vi "GeoData.vi"() -> ()   [LabVIEW 2017]
panel:
  out "StateFIPS":i32[](array[numeric])
  out "EINS":i32[](array[numeric])
  out "StateName":string[](array[string])
  out "County":string[](array[string])
  out "State":string[](array[string])
  out "City":string[](array[string])
  out "Fips":i32[](array[numeric])
  out "Zip":i32[](array[numeric])
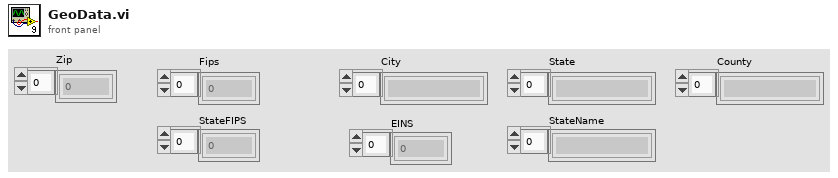
[diagram p1: front panel]
diagram:
  n1 = Spreadsheet String To Array(format string="%s", spreadsheet string="36091\t1001\tVerbena\tAL\tAutauga County\tH1\n36758\t1001\tPlantersville\tAL\tAutauga County\tH1\n36006\t1001\tBillingsley\tAL\tAutauga County\tH1\n36067\t1001\tPrattville\tAL\tAutauga County\tH1\n36701\t1001\tSelma\tAL\tAutauga County\tH1\n36003\t1001\tAutaugaville\tAL\tAutauga County\tH1\n36008\t1001\tBooth\tAL\tAutauga County\tH1\n36068\t1001\tPrattville\tAL\tAutauga County\tH1\n36022\t1001\tDeatsville\tAL\tAutauga County\tH1\n36703\t1001\tSelma\tAL\tAutauga County\tH1\n36749\t1001\tJones\tAL\tAutauga County\tH1\n36066\t1001\tPrattville\tAL\tAutauga County\tH1\n36051\t1001\tMarbury\tAL\tAutauga County\tH1\n36502\t1003\tAtmore\tAL\tBaldwin County\tH1\n36507\t1003\tBay minette\tAL\tBaldwin County\tH1\n36527\t1003\tDaphne\tAL\tBaldwin County\tH1\n36532\t1003\tFairhope\tAL\tBaldwin County\tH1\n36561\t1003\tOrange beach\tAL\tBaldwin County\tH1\n36550\t1003\tLittle river\tAL\tBaldwin County\tH1\n36564\t1003\tPoint clear\tAL\tBaldwin County\tH1\n36579\t1003\tStockton\tAL\tBaldwin County\tH1\n36526\t1003\tDaphne\tAL\tBaldwin County\tH1\n36551\t1003\tLoxley\tAL\tBaldwin County\tH1\n36555\t1003\tMagnolia springs\tAL\tBaldwin County\tH1\n36542\t1003\tGulf shores\tAL\tBaldwin County\tH1\n36567\t1003\tRobertsdale\tAL\tBaldwin County\tH1\n36533\t1003\tFairhope\tAL\tBaldwin County\tH1\n36576\t1003\tSilverhill\tAL\tBaldwin County\tH1\n36580\t1003\tSummerdale\tAL\tBaldwin County\tH1\n36547\t1003\tGulf shores\tAL\tBaldwin County\tH1\n36559\t1003\tMontrose\tAL\tBaldwin County\tH1\n36562\t1003\tPerdido\tAL\tBaldwin County\tH1\n36549\t1003\tLillian\tAL\tBaldwin County\tH1\n36577\t1003\tSpanish fort\tAL\tBaldwin County\tH1\n36511\t1003\tBon secour\tAL\tBaldwin County\tH1\n36530\t1003\tElberta\tAL\tBaldwin County\tH1\n36480\t1003\tUriah\tAL\tBaldwin County\tH1\n36535\t1003\tFoley\tAL\tBaldwin County\tH1\n36574\t1003\tSeminole\tAL\tBaldwin County\tH1\n36536\t1003\tFoley\tAL\tBaldwin County\tH1\n36578\t1003\tStapleton\tAL\tBaldwin County\tH1\n36017\t1005\tClio\tAL\tBarbour County\tH1\n36016\t1005\tClayton\tAL\tBarbour County\tH1\n36317\t1005\tClopton\tAL\tBarbour County\tH1\n36072\t1005\tEufaula\tAL\tBarbour County\tH1\n36311\t1005\tAriton\tAL\tBarbour County\tH1\n36048\t1005\tLouisville\tAL\tBarbour County\tH1\n36053\t1005\tMidway\tAL\tBarbour County\tH1\n36374\t1005\tSkipperville\tAL\tBarbour County\tH1\n36027\t1005\tEufaula\tAL\tBarbour County\tH1\n35115\t1007\tMontevallo\tAL\tBibb County\tH1\n35184\t1007\tWest blocton\tAL\tBibb County\tH1\n36750\t1007\tMaplesville\tAL\tBibb County\tH1\n36756\t1007\tMarion\tAL\tBibb County\tH1\n35074\t1007\tGreen pond\tAL\tBibb County\tH1\n35042\t1007\tCentreville\tAL\tBibb County\tH1\n35111\t1007\tMc calla\tAL\tBibb County\tH1\n35456\t1007\tDuncanville\tAL\tBibb County\tH1\n36792\t1007\tRandolph\tAL\tBibb County\tH1\n35080\t1007\tHelena\tAL\tBibb County\tH1\n35188\t1007\tWoodstock\tAL\tBibb County\tH1\n35034\t1007\tBrent\tAL\tBibb County\tH1\n35035\t1007\tBrierfield\tAL\tBibb County\tH1\n36793\t1007\tLawley\tAL\tBibb County\tH1\n35063\t1009\tEmpire\tAL\tBlount County\tH1\n35146\t1009\tSpringville\tAL\tBlount County\tH1\n35980\t1009\tHorton\tAL\tBlount County\tH1\n35013\t1009\tAllgood\tAL\tBlount County\tH1\n35126\t1009\tPinson\tAL\tBlount County\tH1\n35097\t1009\tLocust fork\tAL\tBlount County\tH1\n35049\t1009\tCleveland\tAL\tBlount County\tH1\n35172\t1009\tTrafford\tAL\tBlount County\tH1\n35957\t1009\tBoaz\tAL\tBlount County\tH1\n35031\t1009\tBlountsville\tAL\tBlount County\tH1\n35133\t1009\tRemlap\tAL\tBlount County\tH1\n35976\t1009\tGuntersville\tAL\tBlount County\tH1\n35016\t1009\tArab\tAL\tBlount County\tH1\n35121\t1009\tOneonta\tAL\tBlount County\tH1\n35079\t1009\tHayden\tAL\tBlount County\tH1\n35180\t1009\tWarrior\tAL\tBlount County\tH1\n35952\t1009\tAltoona\tAL\tBlount County\tH1\n36029\t1011\tFitzpatrick\tAL\tBullock County\tH1\n36052\t1011\tMathews\tAL\tBullock County\tH1\n36089\t1011\tUnion springs\tAL\tBullock County\tH1\n36860\t1011\tHurtsboro\tAL\tBullock County\tH1\n36031\t1011\tFort davis\tAL\tBullock County\tH1\n36081\t1011\tTroy\tAL\tBullock County\tH1\n36053\t1011\tMidway\tAL\tBullock County\tH1\n36005\t1011\tBanks\tAL\tBullock County\tH1\n36830\t1011\tAuburn\tAL\tBullock County\tH1\n36071\t1013\tRutledge\tAL\tButler County\tH1\n36015\t1013\tChapman\tAL\tButler County\tH1\n36042\t1013\tHonoraville\tAL\tButler County\tH1\n36474\t1013\tRed level\tAL\tButler County\tH1\n36033\t1013\tGeorgiana\tAL\tButler County\tH1\n36456\t1013\tMc kenzie\tAL\tButler County\tH1\n36030\t1013\tForest home\tAL\tButler County\tH1\n36032\t1013\tFort deposit\tAL\tButler County\tH1\n36037\t1013\tGreenville\tAL\tButler County\tH1\n36205\t1015\tAnniston\tAL\tCalhoun County\tH1\n36250\t1015\tAlexandria\tAL\tCalhoun County\tH1\n36204\t1015\tAnniston\tAL\tCalhoun County\tH1\n36253\t1015\tBynum\tAL\tCalhoun County\tH1\n35096\t1015\tLincoln\tAL\tCalhoun County\tH1\n35905\t1015\tGadsden\tAL\tCalhoun County\tH1\n36206\t1015\tAnniston\tAL\tCalhoun County\tH1\n36277\t1015\tWeaver\tAL\tCalhoun County\tH1\n36260\t1015\tEastaboga\tAL\tCalhoun County\tH1\n36207\t1015\tAnniston\tAL\tCalhoun County\tH1\n36272\t1015\tPiedmont\tAL\tCalhoun County\tH1\n36202\t1015\tAnniston\tAL\tCalhoun County\tH1\n36265\t1015\tJacksonville\tAL\tCalhoun County\tH1\n36201\t1015\tAnniston\tAL\tCalhoun County\tH1\n36203\t1015\tOxford\tAL\tCalhoun County\tH1\n36257\t1015\tDe armanville\tAL\tCalhoun County\tH1\n36271\t1015\tOhatchee\tAL\tCalhoun County\tH1\n36279\t1015\tWellington\tAL\tCalhoun County\tH1\n36254\t1015\tChoccolocco\tAL\tCalhoun County\tH1\n36854\t1017\tValley\tAL\tChambers County\tH1\n36850\t1017\tCamp hill\tAL\tChambers County\tH1\n36879\t1017\tWaverly\tAL\tChambers County\tH1\n36852\t1017\tCusseta\tAL\tChambers County\tH1\n36276\t1017\tWadley\tAL\tChambers County\tH1\n36274\t1017\tRoanoke\tAL\tChambers County\tH1\n36801\t1017\tOpelika\tAL\tChambers County\tH1\n36863\t1017\tLanett\tAL\tChambers County\tH1\n36862\t1017\tLafayette\tAL\tChambers County\tH1\n36855\t1017\tFive points\tAL\tChambers County\tH1\n35984\t1019\tMentone\tAL\tCherokee County\tH1\n35973\t1019\tGaylesville\tAL\tCherokee County\tH1\n35901\t1019\tGadsden\tAL\tCherokee County\tH1\n36275\t1019\tSpring garden\tAL\tCherokee County\tH1\n35903\t1019\tGadsden\tAL\tCherokee County\tH1\n35983\t1019\tLeesburg\tAL\tCherokee County\tH1\n35959\t1019\tCedar bluff\tAL\tCherokee County\tH1\n35961\t1019\tCollinsville\tAL\tCherokee County\tH1\n35967\t1019\tFort payne\tAL\tCherokee County\tH1\n36272\t1019\tPiedmont\tAL\tCherokee County\tH1\n35960\t1019\tCentre\tAL\tCherokee County\tH1\n35115\t1021\tMontevallo\tAL\tChilton County\tH1\n36091\t1021\tVerbena\tAL\tChilton County\tH1\n36758\t1021\tPlantersville\tAL\tChilton County\tH1\n36790\t1021\tStanton\tAL\tChilton County\tH1\n36006\t1021\tBillingsley\tAL\tChilton County\tH1\n36750\t1021\tMaplesville\tAL\tChilton County\tH1\n35045\t1021\tClanton\tAL\tChilton County\tH1\n36792\t1021\tRandolph\tAL\tChilton County\tH1\n35040\t1021\tCalera\tAL\tChilton County\tH1\n35046\t1021\tClanton\tAL\tChilton County\tH1\n35171\t1021\tThorsby\tAL\tChilton County\tH1\n36051\t1021\tMarbury\tAL\tChilton County\tH1\n35085\t1021\tJemison\tAL\tChilton County\tH1\n36793\t1021\tLawley\tAL\tChilton County\tH1\n36915\t1023\tNeedham\tAL\tChoctaw County\tH1\n36919\t1023\tSilas\tAL\tChoctaw County\tH1\n36910\t1023\tJachin\tAL\tChoctaw County\tH1\n36916\t1023\tPennington\tAL\tChoctaw County\tH1\n36908\t1023\tGilbertown\tAL\tChoctaw County\tH1\n36913\t1023\tMelvin\tAL\tChoctaw County\tH1\n36912\t1023\tLisman\tAL\tChoctaw County\tH1\n36921\t1023\tToxey\tAL\tChoctaw County\tH1\n36558\t1023\tMillry\tAL\tChoctaw County\tH1\n36904\t1023\tButler\tAL\tChoctaw County\tH1\n36922\t1023\tWard\tAL\tChoctaw County\tH1\n36540\t1025\tGainestown\tAL\tClarke County\tH1\n36524\t1025\tCoffeeville\tAL\tClarke County\tH1\n36751\t1025\tLower peach tree\tAL\tClarke County\tH1\n36727\t1025\tCampbell\tAL\tClarke County\tH1\n36545\t1025\tJackson\tAL\tClarke County\tH1\n36446\t1025\tFulton\tAL\tClarke County\tH1\n36451\t1025\tGrove hill\tAL\tClarke County\tH1\n36436\t1025\tDickinson\tAL\tClarke County\tH1\n36784\t1025\tThomasville\tAL\tClarke County\tH1\n36482\t1025\tWhatley\tAL\tClarke County\tH1\n36251\t1027\tAshland\tAL\tClay County\tH1\n35089\t1027\tKellyton\tAL\tClay County\tH1\n36266\t1027\tLineville\tAL\tClay County\tH1\n36267\t1027\tMillerville\tAL\tClay County\tH1\n36256\t1027\tDaviston\tAL\tClay County\tH1\n36258\t1027\tDelta\tAL\tClay County\tH1\n36255\t1027\tCragford\tAL\tClay County\tH1\n35072\t1027\tGoodwater\tAL\tClay County\tH1\n35160\t1027\tTalladega\tAL\tClay County\tH1\n36276\t1027\tWadley\tAL\tClay County\tH1\n36268\t1027\tMunford\tAL\tClay County\tH1\n35082\t1027\tHollins\tAL\tClay County\tH1\n36264\t1029\tHeflin\tAL\tCleburne County\tH1\n36269\t1029\tMuscadine\tAL\tCleburne County\tH1\n36258\t1029\tDelta\tAL\tCleburne County\tH1\n36207\t1029\tAnniston\tAL\tCleburne County\tH1\n36272\t1029\tPiedmont\tAL\tCleburne County\tH1\n36262\t1029\tFruithurst\tAL\tCleburne County\tH1\n36273\t1029\tRanburne\tAL\tCleburne County\tH1\n36261\t1029\tEdwardsville\tAL\tCleburne County\tH1\n36268\t1029\tMunford\tAL\tCleburne County\tH1\n36323\t1031\tElba\tAL\tCoffee County\tH1\n36360\t1031\tOzark\tAL\tCoffee County\tH1\n36079\t1031\tTroy\tAL\tCoffee County\tH1\n36322\t1031\tDaleville\tAL\tCoffee County\tH1\n36311\t1031\tAriton\tAL\tCoffee County\tH1\n36453\t1031\tKinston\tAL\tCoffee County\tH1\n36009\t1031\tBrantley\tAL\tCoffee County\tH1\n36351\t1031\tNew brockton\tAL\tCoffee County\tH1\n36010\t1031\tBrundidge\tAL\tCoffee County\tH1\n36330\t1031\tEnterprise\tAL\tCoffee County\tH1\n36316\t1031\tChancellor\tAL\tCoffee County\tH1\n36034\t1031\tGlenwood\tAL\tCoffee County\tH1\n36467\t1031\tOpp\tAL\tCoffee County\tH1\n36346\t1031\tJack\tAL\tCoffee County\tH1\n36477\t1031\tSamson\tAL\tCoffee County\tH1\n36318\t1031\tCoffee springs\tAL\tCoffee County\tH1\n35672\t1033\tTown creek\tAL\tColbert County\tH1\n35646\t1033\tLeighton\tAL\tColbert County\tH1\n35616\t1033\tCherokee\tAL\tColbert County\tH1\n35661\t1033\tMuscle shoals\tAL\tColbert County\tH1\n35674\t1033\tTuscumbia\tAL\tColbert County\tH1\n35654\t1033\tRussellville\tAL\tColbert County\tH1\n35660\t1033\tSheffield\tAL\tColbert County\tH1\n35653\t1033\tRussellville\tAL\tColbert County\tH1\n35582\t1033\tRed bay\tAL\tColbert County\tH1\n36502\t1035\tAtmore\tAL\tConecuh County\tH1\n36474\t1035\tRed level\tAL\tConecuh County\tH1\n36033\t1035\tGeorgiana\tAL\tConecuh County\tH1\n36456\t1035\tMc kenzie\tAL\tConecuh County\tH1\n36473\t1035\tRange\tAL\tConecuh County\tH1\n36330\t1035\tEnterprise\tAL\tConecuh County\tH1\n36471\t1035\tPeterman\tAL\tConecuh County\tH1\n36454\t1035\tLenox\tAL\tConecuh County\tH1\n36460\t1035\tMonroeville\tAL\tConecuh County\tH1\n36401\t1035\tEvergreen\tAL\tConecuh County\tH1\n36421\t1035\tAndalusia\tAL\tConecuh County\tH1\n36426\t1035\tBrewton\tAL\tConecuh County\tH1\n36432\t1035\tCastleberry\tAL\tConecuh County\tH1\n36475\t1035\tRepton\tAL\tConecuh County\tH1\n36768\t1035\tPine apple\tAL\tConecuh County\tH1\n35151\t1037\tSylacauga\tAL\tCoosa County\tH1\n35010\t1037\tAlexander city\tAL\tCoosa County\tH1\n35183\t1037\tWeogufka\tAL\tCoosa County\tH1\n35089\t1037\tKellyton\tAL\tCoosa County\tH1\n36026\t1037\tEquality\tAL\tCoosa County\tH1\n35150\t1037\tSylacauga\tAL\tCoosa County\tH1\n35072\t1037\tGoodwater\tAL\tCoosa County\tH1\n35136\t1037\tRockford\tAL\tCoosa County\tH1\n35046\t1037\tClanton\tAL\tCoosa County\tH1\n36080\t1037\tTitus\tAL\tCoosa County\tH1\n36476\t1039\tRiver falls\tAL\tCovington County\tH1\n36028\t1039\tDozier\tAL\tCovington County\tH1\n36474\t1039\tRed level\tAL\tCovington County\tH1\n36453\t1039\tKinston\tAL\tCovington County\tH1\n36456\t1039\tMc kenzie\tAL\tCovington County\tH1\n36038\t1039\tGantt\tAL\tCovington County\tH1\n36442\t1039\tFlorala\tAL\tCovington County\tH1\n36455\t1039\tLockhart\tAL\tCovington County\tH1\n36420\t1039\tAndalusia\tAL\tCovington County\tH1\n36401\t1039\tEvergreen\tAL\tCovington County\tH1\n36421\t1039\tAndalusia\tAL\tCovington County\tH1\n36467\t1039\tOpp\tAL\tCovington County\tH1\n36483\t1039\tWing\tAL\tCovington County\tH1\n36477\t1039\tSamson\tAL\tCovington County\tH1\n36323\t1041\tElba\tAL\tCrenshaw County\tH1\n36028\t1041\tDozier\tAL\tCrenshaw County\tH1\n36071\t1041\tRutledge\tAL\tCrenshaw County\tH1\n36042\t1041\tHonoraville\tAL\tCrenshaw County\tH1\n36009\t1041\tBrantley\tAL\tCrenshaw County\tH1\n36049\t1041\tLuverne\tAL\tCrenshaw County\tH1\n36041\t1041\tHighland home\tAL\tCrenshaw County\tH1\n36032\t1041\tFort deposit\tAL\tCrenshaw County\tH1\n36034\t1041\tGlenwood\tAL\tCrenshaw County\tH1\n36035\t1041\tGoshen\tAL\tCrenshaw County\tH1\n36467\t1041\tOpp\tAL\tCrenshaw County\tH1\n36037\t1041\tGreenville\tAL\tCrenshaw County\tH1\n36036\t1041\tGrady\tAL\tCrenshaw County\tH1\n36046\t1041\tLapine\tAL\tCrenshaw County\tH1\n35619\t1043\tDanville\tAL\tCullman County\tH1\n35541\t1043\tArley\tAL\tCullman County\tH1\n35057\t1043\tCullman\tAL\tCullman County\tH1\n35033\t1043\tBremen\tAL\tCullman County\tH1\n35055\t1043\tCullman\tAL\tCullman County\tH1\n35058\t1043\tCullman\tAL\tCullman County\tH1\n35077\t1043\tHanceville\tAL\tCullman County\tH1\n35070\t1043\tGarden city\tAL\tCullman County\tH1\n35087\t1043\tJoppa\tAL\tCullman County\tH1\n35083\t1043\tHolly pond\tAL\tCullman County\tH1\n35098\t1043\tLogan\tAL\tCullman County\tH1\n35976\t1043\tGuntersville\tAL\tCullman County\tH1\n35056\t1043\tCullman\tAL\tCullman County\tH1\n35053\t1043\tCrane hill\tAL\tCullman County\tH1\n35019\t1043\tBaileyton\tAL\tCullman County\tH1\n35016\t1043\tArab\tAL\tCullman County\tH1\n35179\t1043\tVinemont\tAL\tCullman County\tH1\n35540\t1043\tAddison\tAL\tCullman County\tH1\n35621\t1043\tEva\tAL\tCullman County\tH1\n35622\t1043\tFalkville\tAL\tCullman County\tH1\n35670\t1043\tSomerville\tAL\tCullman County\tH1\n36360\t1045\tOzark\tAL\tDale County\tH1\n36317\t1045\tClopton\tAL\tDale County\tH1\n36322\t1045\tDaleville\tAL\tDale County\tH1\n36361\t1045\tOzark\tAL\tDale County\tH1\n36371\t1045\tPinckard\tAL\tDale County\tH1\n36311\t1045\tAriton\tAL\tDale County\tH1\n36362\t1045\tFort rucker\tAL\tDale County\tH1\n36345\t1045\tHeadland\tAL\tDale County\tH1\n36010\t1045\tBrundidge\tAL\tDale County\tH1\n36330\t1045\tEnterprise\tAL\tDale County\tH1\n36352\t1045\tNewton\tAL\tDale County\tH1\n36374\t1045\tSkipperville\tAL\tDale County\tH1\n36303\t1045\tDothan\tAL\tDale County\tH1\n36353\t1045\tNewville\tAL\tDale County\tH1\n36350\t1045\tMidland city\tAL\tDale County\tH1\n36758\t1047\tPlantersville\tAL\tDallas County\tH1\n36773\t1047\tSafford\tAL\tDallas County\tH1\n36701\t1047\tSelma\tAL\tDallas County\tH1\n36785\t1047\tTyler\tAL\tDallas County\tH1\n36703\t1047\tSelma\tAL\tDallas County\tH1\n36775\t1047\tSardis\tAL\tDallas County\tH1\n36761\t1047\tMinter\tAL\tDallas County\tH1\n36749\t1047\tJones\tAL\tDallas County\tH1\n36767\t1047\tOrrville\tAL\tDallas County\tH1\n36759\t1047\tMarion junction\tAL\tDallas County\tH1\n35968\t1049\tFort payne\tAL\tDeKalb County\tH1\n35984\t1049\tMentone\tAL\tDeKalb County\tH1\n35765\t1049\tPisgah\tAL\tDeKalb County\tH1\n35954\t1049\tAttalla\tAL\tDeKalb County\tH1\n35983\t1049\tLeesburg\tAL\tDeKalb County\tH1\n35966\t1049\tFlat rock\tAL\tDeKalb County\tH1\n35975\t1049\tGroveoak\tAL\tDeKalb County\tH1\n35957\t1049\tBoaz\tAL\tDeKalb County\tH1\n35959\t1049\tCedar bluff\tAL\tDeKalb County\tH1\n35978\t1049\tHenagar\tAL\tDeKalb County\tH1\n35988\t1049\tSylvania\tAL\tDeKalb County\tH1\n35951\t1049\tAlbertville\tAL\tDeKalb County\tH1\n35961\t1049\tCollinsville\tAL\tDeKalb County\tH1\n35967\t1049\tFort payne\tAL\tDeKalb County\tH1\n35956\t1049\tBoaz\tAL\tDeKalb County\tH1\n35981\t1049\tIder\tAL\tDeKalb County\tH1\n35974\t1049\tGeraldine\tAL\tDeKalb County\tH1\n35979\t1049\tHigdon\tAL\tDeKalb County\tH1\n35989\t1049\tValley head\tAL\tDeKalb County\tH1\n35963\t1049\tDawson\tAL\tDeKalb County\tH1\n35962\t1049\tCrossville\tAL\tDeKalb County\tH1\n35971\t1049\tFyffe\tAL\tDeKalb County\tH1\n35986\t1049\tRainsville\tAL\tDeKalb County\tH1\n35771\t1049\tSection\tAL\tDeKalb County\tH1\n36024\t1051\tEclectic\tAL\tElmore County\tH1\n35010\t1051\tAlexander city\tAL\tElmore County\tH1\n36078\t1051\tTallassee\tAL\tElmore County\tH1\n36067\t1051\tPrattville\tAL\tElmore County\tH1\n36092\t1051\tWetumpka\tAL\tElmore County\tH1\n36093\t1051\tWetumpka\tAL\tElmore County\tH1\n36026\t1051\tEquality\tAL\tElmore County\tH1\n36054\t1051\tMillbrook\tAL\tElmore County\tH1\n35136\t1051\tRockford\tAL\tElmore County\tH1\n36025\t1051\tElmore\tAL\tElmore County\tH1\n36022\t1051\tDeatsville\tAL\tElmore County\tH1\n36066\t1051\tPrattville\tAL\tElmore County\tH1\n36051\t1051\tMarbury\tAL\tElmore County\tH1\n36020\t1051\tCoosada\tAL\tElmore County\tH1\n36080\t1051\tTitus\tAL\tElmore County\tH1\n36502\t1053\tAtmore\tAL\tEscambia County\tH1\n36441\t1053\tFlomaton\tAL\tEscambia County\tH1\n36420\t1053\tAndalusia\tAL\tEscambia County\tH1\n36426\t1053\tBrewton\tAL\tEscambia County\tH1\n36432\t1053\tCastleberry\tAL\tEscambia County\tH1\n36475\t1053\tRepton\tAL\tEscambia County\tH1\n36483\t1053\tWing\tAL\tEscambia County\tH1\n36562\t1053\tPerdido\tAL\tEscambia County\tH1\n36543\t1053\tHuxford\tAL\tEscambia County\tH1\n36503\t1053\tAtmore\tAL\tEscambia County\tH1\n35901\t1055\tGadsden\tAL\tEtowah County\tH1\n35954\t1055\tAttalla\tAL\tEtowah County\tH1\n35903\t1055\tGadsden\tAL\tEtowah County\tH1\n35907\t1055\tGadsden\tAL\tEtowah County\tH1\n35905\t1055\tGadsden\tAL\tEtowah County\tH1\n35904\t1055\tGadsden\tAL\tEtowah County\tH1\n35957\t1055\tBoaz\tAL\tEtowah County\tH1\n35961\t1055\tCollinsville\tAL\tEtowah County\tH1\n35972\t1055\tGallant\tAL\tEtowah County\tH1\n35956\t1055\tBoaz\tAL\tEtowah County\tH1\n36272\t1055\tPiedmont\tAL\tEtowah County\tH1\n35902\t1055\tGadsden\tAL\tEtowah County\tH1\n35990\t1055\tWalnut grove\tAL\tEtowah County\tH1\n35121\t1055\tOneonta\tAL\tEtowah County\tH1\n35952\t1055\tAltoona\tAL\tEtowah County\tH1\n35906\t1055\tRainbow city\tAL\tEtowah County\tH1\n36271\t1055\tOhatchee\tAL\tEtowah County\tH1\n35554\t1057\tEldridge\tAL\tFayette County\tH1\n35594\t1057\tWinfield\tAL\tFayette County\tH1\n35546\t1057\tBerry\tAL\tFayette County\tH1\n35549\t1057\tCarbon hill\tAL\tFayette County\tH1\n35579\t1057\tOakman\tAL\tFayette County\tH1\n35563\t1057\tGuin\tAL\tFayette County\tH1\n35542\t1057\tBankston\tAL\tFayette County\tH1\n35545\t1057\tBelk\tAL\tFayette County\tH1\n35574\t1057\tKennedy\tAL\tFayette County\tH1\n35555\t1057\tFayette\tAL\tFayette County\tH1\n35559\t1057\tGlen allen\tAL\tFayette County\tH1\n35585\t1059\tSpruce pine\tAL\tFranklin County\tH1\n35593\t1059\tVina\tAL\tFranklin County\tH1\n35581\t1059\tPhil campbell\tAL\tFranklin County\tH1\n35616\t1059\tCherokee\tAL\tFranklin County\tH1\n35674\t1059\tTuscumbia\tAL\tFranklin County\tH1\n35565\t1059\tHaleyville\tAL\tFranklin County\tH1\n35564\t1059\tHackleburg\tAL\tFranklin County\tH1\n35651\t1059\tMount hope\tAL\tFranklin County\tH1\n35654\t1059\tRussellville\tAL\tFranklin County\tH1\n35571\t1059\tHodges\tAL\tFranklin County\tH1\n35653\t1059\tRussellville\tAL\tFranklin County\tH1\n35582\t1059\tRed bay\tAL\tFranklin County\tH1\n36305\t1061\tDothan\tAL\tGeneva County\tH1\n36314\t1061\tBlack\tAL\tGeneva County\tH1\n36322\t1061\tDaleville\tAL\tGeneva County\tH1\n36375\t1061\tSlocomb\tAL\tGeneva County\tH1\n36453\t1061\tKinston\tAL\tGeneva County\tH1\n36340\t1061\tGeneva\tAL\tGeneva County\tH1\n36344\t1061\tHartford\tAL\tGeneva County\tH1\n36316\t1061\tChancellor\tAL\tGeneva County\tH1\n36442\t1061\tFlorala\tAL\tGeneva County\tH1\n36352\t1061\tNewton\tAL\tGeneva County\tH1\n36301\t1061\tDothan\tAL\tGeneva County\tH1\n36467\t1061\tOpp\tAL\tGeneva County\tH1\n36349\t1061\tMalvern\tAL\tGeneva County\tH1\n36477\t1061\tSamson\tAL\tGeneva County\tH1\n36318\t1061\tCoffee springs\tAL\tGeneva County\tH1\n36313\t1061\tBellwood\tAL\tGeneva County\tH1\n35480\t1063\tRalph\tAL\tGreene County\tH1\n35448\t1063\tClinton\tAL\tGreene County\tH1\n35464\t1063\tGainesville\tAL\tGreene County\tH1\n35443\t1063\tBoligee\tAL\tGreene County\tH1\n35463\t1063\tFosters\tAL\tGreene County\tH1\n35469\t1063\tKnoxville\tAL\tGreene County\tH1\n35491\t1063\tWest greene\tAL\tGreene County\tH1\n35462\t1063\tEutaw\tAL\tGreene County\tH1\n36740\t1063\tForkland\tAL\tGreene County\tH1\n36744\t1065\tGreensboro\tAL\tHale County\tH1\n36786\t1065\tUniontown\tAL\tHale County\tH1\n36756\t1065\tMarion\tAL\tHale County\tH1\n36765\t1065\tNewbern\tAL\tHale County\tH1\n35441\t1065\tAkron\tAL\tHale County\tH1\n35474\t1065\tMoundville\tAL\tHale County\tH1\n36742\t1065\tGallion\tAL\tHale County\tH1\n36776\t1065\tSawyerville\tAL\tHale County\tH1\n36738\t1065\tFaunsdale\tAL\tHale County\tH1\n36317\t1067\tClopton\tAL\tHenry County\tH1\n36373\t1067\tShorterville\tAL\tHenry County\tH1\n36319\t1067\tColumbia\tAL\tHenry County\tH1\n36345\t1067\tHeadland\tAL\tHenry County\tH1\n36303\t1067\tDothan\tAL\tHenry County\tH1\n36310\t1067\tAbbeville\tAL\tHenry County\tH1\n36353\t1067\tNewville\tAL\tHenry County\tH1\n36350\t1067\tMidland city\tAL\tHenry County\tH1\n36320\t1069\tCottonwood\tAL\tHouston County\tH1\n36305\t1069\tDothan\tAL\tHouston County\tH1\n36312\t1069\tAshford\tAL\tHouston County\tH1\n36375\t1069\tSlocomb\tAL\tHouston County\tH1\n36319\t1069\tColumbia\tAL\tHouston County\tH1\n36345\t1069\tHeadland\tAL\tHouston County\tH1\n36376\t1069\tWebb\tAL\tHouston County\tH1\n36352\t1069\tNewton\tAL\tHouston County\tH1\n36302\t1069\tDothan\tAL\tHouston County\tH1\n36301\t1069\tDothan\tAL\tHouston County\tH1\n36303\t1069\tDothan\tAL\tHouston County\tH1\n36321\t1069\tCowarts\tAL\tHouston County\tH1\n36343\t1069\tGordon\tAL\tHouston County\tH1\n36370\t1069\tPansey\tAL\tHouston County\tH1\n36350\t1069\tMidland city\tAL\tHouston County\tH1\n35751\t1071\tHollytree\tAL\tJackson County\tH1\n35752\t1071\tHollywood\tAL\tJackson County\tH1\n35765\t1071\tPisgah\tAL\tJackson County\tH1\n35745\t1071\tEstillfork\tAL\tJackson County\tH1\n35776\t1071\tWoodville\tAL\tJackson County\tH1\n35966\t1071\tFlat rock\tAL\tJackson County\tH1\n35769\t1071\tScottsboro\tAL\tJackson County\tH1\n35978\t1071\tHenagar\tAL\tJackson County\tH1\n35772\t1071\tStevenson\tAL\tJackson County\tH1\n35768\t1071\tScottsboro\tAL\tJackson County\tH1\n35748\t1071\tGurley\tAL\tJackson County\tH1\n35774\t1071\tTrenton\tAL\tJackson County\tH1\n35958\t1071\tBryant\tAL\tJackson County\tH1\n35740\t1071\tBridgeport\tAL\tJackson County\tH1\n35766\t1071\tPrinceton\tAL\tJackson County\tH1\n35979\t1071\tHigdon\tAL\tJackson County\tH1\n35744\t1071\tDutton\tAL\tJackson County\tH1\n35764\t1071\tPaint rock\tAL\tJackson County\tH1\n35971\t1071\tFyffe\tAL\tJackson County\tH1\n35746\t1071\tFackler\tAL\tJackson County\tH1\n35755\t1071\tLangston\tAL\tJackson County\tH1\n35771\t1071\tSection\tAL\tJackson County\tH1\n35022\t1073\tBessemer\tAL\tJefferson County\tH1\n35130\t1073\tQuinton\tAL\tJefferson County\tH1\n35208\t1073\tBirmingham\tAL\tJefferson County\tH1\n35242\t1073\tBirmingham\tAL\tJefferson County\tH1\n35244\t1073\tBirmingham\tAL\tJefferson County\tH1\n35221\t1073\tBirmingham\tAL\tJefferson County\tH1\n35224\t1073\tBirmingham\tAL\tJefferson County\tH1\n35253\t1073\tBirmingham\tAL\tJefferson County\tH1\n35218\t1073\tBirmingham\tAL\tJefferson County\tH1\n35243\t1073\tBirmingham\tAL\tJefferson County\tH1\n35060\t1073\tDocena\tAL\tJefferson County\tH1\n35123\t1073\tPalmerdale\tAL\tJefferson County\tH1\n35181\t1073\tWatson\tAL\tJefferson County\tH1\n35063\t1073\tEmpire\tAL\tJefferson County\tH1\n35094\t1073\tLeeds\tAL\tJefferson County\tH1\n35005\t1073\tAdamsville\tAL\tJefferson County\tH1\n35146\t1073\tSpringville\tAL\tJefferson County\tH1\n35203\t1073\tBirmingham\tAL\tJefferson County\tH1\n35117\t1073\tMount olive\tAL\tJefferson County\tH1\n35211\t1073\tBirmingham\tAL\tJefferson County\tH1\n35222\t1073\tBirmingham\tAL\tJefferson County\tH1\n35216\t1073\tBirmingham\tAL\tJefferson County\tH1\n35091\t1073\tKimberly\tAL\tJefferson County\tH1\n35231\t1073\tBirmingham\tAL\tJefferson County\tH1\n35021\t1073\tBessemer\tAL\tJefferson County\tH1\n35036\t1073\tBrookside\tAL\tJefferson County\tH1\n35294\t1073\tBirmingham\tAL\tJefferson County\tH1\n35254\t1073\tBirmingham\tAL\tJefferson County\tH1\n35293\t1073\tBirmingham\tAL\tJefferson County\tH1\n35061\t1073\tDolomite\tAL\tJefferson County\tH1\n35064\t1073\tFairfield\tAL\tJefferson County\tH1\n35126\t1073\tPinson\tAL\tJefferson County\tH1\n35127\t1073\tPleasant grove\tAL\tJefferson County\tH1\n35206\t1073\tBirmingham\tAL\tJefferson County\tH1\n35210\t1073\tBirmingham\tAL\tJefferson County\tH1\n35202\t1073\tBirmingham\tAL\tJefferson County\tH1\n35214\t1073\tBirmingham\tAL\tJefferson County\tH1\n35215\t1073\tBirmingham\tAL\tJefferson County\tH1\n35233\t1073\tBirmingham\tAL\tJefferson County\tH1\n35444\t1073\tBrookwood\tAL\tJefferson County\tH1\n35236\t1073\tBirmingham\tAL\tJefferson County\tH1\n35023\t1073\tBessemer\tAL\tJefferson County\tH1\n35073\t1073\tGraysville\tAL\tJefferson County\tH1\n35004\t1073\tMoody\tAL\tJefferson County\tH1\n35172\t1073\tTrafford\tAL\tJefferson County\tH1\n35111\t1073\tMc calla\tAL\tJefferson County\tH1\n35118\t1073\tMulga\tAL\tJefferson County\tH1\n35048\t1073\tClay\tAL\tJefferson County\tH1\n35220\t1073\tBirmingham\tAL\tJefferson County\tH1\n35219\t1073\tBirmingham\tAL\tJefferson County\tH1\n35139\t1073\tSayre\tAL\tJefferson County\tH1\n35068\t1073\tFultondale\tAL\tJefferson County\tH1\n35006\t1073\tAdger\tAL\tJefferson County\tH1\n35173\t1073\tTrussville\tAL\tJefferson County\tH1\n35205\t1073\tBirmingham\tAL\tJefferson County\tH1\n35209\t1073\tBirmingham\tAL\tJefferson County\tH1\n35235\t1073\tBirmingham\tAL\tJefferson County\tH1\n35234\t1073\tBirmingham\tAL\tJefferson County\tH1\n35260\t1073\tBirmingham\tAL\tJefferson County\tH1\n35261\t1073\tBirmingham\tAL\tJefferson County\tH1\n35295\t1073\tBirmingham\tAL\tJefferson County\tH1\n35020\t1073\tBessemer\tAL\tJefferson County\tH1\n35133\t1073\tRemlap\tAL\tJefferson County\tH1\n35116\t1073\tMorris\tAL\tJefferson County\tH1\n35255\t1073\tBirmingham\tAL\tJefferson County\tH1\n35223\t1073\tBirmingham\tAL\tJefferson County\tH1\n35217\t1073\tBirmingham\tAL\tJefferson County\tH1\n35285\t1073\tBirmingham\tAL\tJefferson County\tH1\n35270\t1073\tBirmingham\tAL\tJefferson County\tH1\n35142\t1073\tShannon\tAL\tJefferson County\tH1\n35249\t1073\tBirmingham\tAL\tJefferson County\tH1\n35080\t1073\tHelena\tAL\tJefferson County\tH1\n35071\t1073\tGardendale\tAL\tJefferson County\tH1\n35148\t1073\tSumiton\tAL\tJefferson County\tH1\n35213\t1073\tBirmingham\tAL\tJefferson County\tH1\n35212\t1073\tBirmingham\tAL\tJefferson County\tH1\n35228\t1073\tBirmingham\tAL\tJefferson County\tH1\n35259\t1073\tBirmingham\tAL\tJefferson County\tH1\n35119\t1073\tNew castle\tAL\tJefferson County\tH1\n35062\t1073\tDora\tAL\tJefferson County\tH1\n35079\t1073\tHayden\tAL\tJefferson County\tH1\n35204\t1073\tBirmingham\tAL\tJefferson County\tH1\n35207\t1073\tBirmingham\tAL\tJefferson County\tH1\n35201\t1073\tBirmingham\tAL\tJefferson County\tH1\n35180\t1073\tWarrior\tAL\tJefferson County\tH1\n35226\t1073\tBirmingham\tAL\tJefferson County\tH1\n35266\t1073\tBirmingham\tAL\tJefferson County\tH1\n35015\t1073\tAlton\tAL\tJefferson County\tH1\n35232\t1073\tBirmingham\tAL\tJefferson County\tH1\n35229\t1073\tBirmingham\tAL\tJefferson County\tH1\n35576\t1075\tMillport\tAL\tLamar County\tH1\n35586\t1075\tSulligent\tAL\tLamar County\tH1\n35592\t1075\tVernon\tAL\tLamar County\tH1\n35563\t1075\tGuin\tAL\tLamar County\tH1\n35570\t1075\tHamilton\tAL\tLamar County\tH1\n35544\t1075\tBeaverton\tAL\tLamar County\tH1\n35574\t1075\tKennedy\tAL\tLamar County\tH1\n35555\t1075\tFayette\tAL\tLamar County\tH1\n35552\t1075\tDetroit\tAL\tLamar County\tH1\n35614\t1077\tAthens\tAL\tLauderdale County\tH1\n35677\t1077\tWaterloo\tAL\tLauderdale County\tH1\n35630\t1077\tFlorence\tAL\tLauderdale County\tH1\n35634\t1077\tFlorence\tAL\tLauderdale County\tH1\n35633\t1077\tFlorence\tAL\tLauderdale County\tH1\n35648\t1077\tLexington\tAL\tLauderdale County\tH1\n35631\t1077\tFlorence\tAL\tLauderdale County\tH1\n35610\t1077\tAnderson\tAL\tLauderdale County\tH1\n35645\t1077\tKillen\tAL\tLauderdale County\tH1\n35632\t1077\tFlorence\tAL\tLauderdale County\tH1\n35652\t1077\tRogersville\tAL\tLauderdale County\tH1\n35617\t1077\tCloverdale\tAL\tLauderdale County\tH1\n35619\t1079\tDanville\tAL\tLawrence County\tH1\n35672\t1079\tTown creek\tAL\tLawrence County\tH1\n35650\t1079\tMoulton\tAL\tLawrence County\tH1\n35618\t1079\tCourtland\tAL\tLawrence County\tH1\n35673\t1079\tTrinity\tAL\tLawrence County\tH1\n35651\t1079\tMount hope\tAL\tLawrence County\tH1\n35603\t1079\tDecatur\tAL\tLawrence County\tH1\n35654\t1079\tRussellville\tAL\tLawrence County\tH1\n35540\t1079\tAddison\tAL\tLawrence County\tH1\n35643\t1079\tHillsboro\tAL\tLawrence County\tH1\n36874\t1081\tSalem\tAL\tLee County\tH1\n36877\t1081\tSmiths station\tAL\tLee County\tH1\n36849\t1081\tAuburn university\tAL\tLee County\tH1\n36804\t1081\tOpelika\tAL\tLee County\tH1\n36832\t1081\tAuburn\tAL\tLee County\tH1\n36854\t1081\tValley\tAL\tLee County\tH1\n36850\t1081\tCamp hill\tAL\tLee County\tH1\n36879\t1081\tWaverly\tAL\tLee County\tH1\n36866\t1081\tNotasulga\tAL\tLee County\tH1\n36852\t1081\tCusseta\tAL\tLee County\tH1\n36867\t1081\tPhenix city\tAL\tLee County\tH1\n36830\t1081\tAuburn\tAL\tLee County\tH1\n36801\t1081\tOpelika\tAL\tLee County\tH1\n36870\t1081\tPhenix city\tAL\tLee County\tH1\n36803\t1081\tOpelika\tAL\tLee County\tH1\n36831\t1081\tAuburn\tAL\tLee County\tH1\n36865\t1081\tLoachapoka\tAL\tLee County\tH1\n35614\t1083\tAthens\tAL\tLimestone County\tH1\n35749\t1083\tHarvest\tAL\tLimestone County\tH1\n35620\t1083\tElkmont\tAL\tLimestone County\tH1\n35773\t1083\tToney\tAL\tLimestone County\tH1\n35612\t1083\tAthens\tAL\tLimestone County\tH1\n35739\t1083\tArdmore\tAL\tLimestone County\tH1\n35615\t1083\tBelle mina\tAL\tLimestone County\tH1\n35649\t1083\tMooresville\tAL\tLimestone County\tH1\n35756\t1083\tMadison\tAL\tLimestone County\tH1\n35757\t1083\tMadison\tAL\tLimestone County\tH1\n35647\t1083\tLester\tAL\tLimestone County\tH1\n35613\t1083\tAthens\tAL\tLimestone County\tH1\n35671\t1083\tTanner\tAL\tLimestone County\tH1\n35742\t1083\tCapshaw\tAL\tLimestone County\tH1\n35610\t1083\tAnderson\tAL\tLimestone County\tH1\n35611\t1083\tAthens\tAL\tLimestone County\tH1\n35652\t1083\tRogersville\tAL\tLimestone County\tH1\n36043\t1085\tHope hull\tAL\tLowndes County\tH1\n36752\t1085\tLowndesboro\tAL\tLowndes County\tH1\n36047\t1085\tLetohatchee\tAL\tLowndes County\tH1\n36701\t1085\tSelma\tAL\tLowndes County\tH1\n36040\t1085\tHayneville\tAL\tLowndes County\tH1\n36785\t1085\tTyler\tAL\tLowndes County\tH1\n36041\t1085\tHighland home\tAL\tLowndes County\tH1\n36032\t1085\tFort deposit\tAL\tLowndes County\tH1\n36775\t1085\tSardis\tAL\tLowndes County\tH1\n36761\t1085\tMinter\tAL\tLowndes County\tH1\n36039\t1087\tHardaway\tAL\tMacon County\tH1\n36029\t1087\tFitzpatrick\tAL\tMacon County\tH1\n36089\t1087\tUnion springs\tAL\tMacon County\tH1\n36078\t1087\tTallassee\tAL\tMacon County\tH1\n36013\t1087\tCecil\tAL\tMacon County\tH1\n36804\t1087\tOpelika\tAL\tMacon County\tH1\n36860\t1087\tHurtsboro\tAL\tMacon County\tH1\n36087\t1087\tTuskegee institute\tAL\tMacon County\tH1\n36832\t1087\tAuburn\tAL\tMacon County\tH1\n36075\t1087\tShorter\tAL\tMacon County\tH1\n36088\t1087\tTuskegee institute\tAL\tMacon County\tH1\n36879\t1087\tWaverly\tAL\tMacon County\tH1\n36866\t1087\tNotasulga\tAL\tMacon County\tH1\n36083\t1087\tTuskegee\tAL\tMacon County\tH1\n36830\t1087\tAuburn\tAL\tMacon County\tH1\n35803\t1089\tHuntsville\tAL\tMadison County\tH1\n35749\t1089\tHarvest\tAL\tMadison County\tH1\n35760\t1089\tNew hope\tAL\tMadison County\tH1\n35897\t1089\tHuntsville\tAL\tMadison County\tH1\n35810\t1089\tHuntsville\tAL\tMadison County\tH1\n35808\t1089\tHuntsville\tAL\tMadison County\tH1\n35776\t1089\tWoodville\tAL\tMadison County\tH1\n35816\t1089\tHuntsville\tAL\tMadison County\tH1\n35801\t1089\tHuntsville\tAL\tMadison County\tH1\n35773\t1089\tToney\tAL\tMadison County\tH1\n35894\t1089\tHuntsville\tAL\tMadison County\tH1\n35811\t1089\tHuntsville\tAL\tMadison County\tH1\n35741\t1089\tBrownsboro\tAL\tMadison County\tH1\n35739\t1089\tArdmore\tAL\tMadison County\tH1\n35763\t1089\tOwens cross roads\tAL\tMadison County\tH1\n35812\t1089\tHuntsville\tAL\tMadison County\tH1\n35895\t1089\tHuntsville\tAL\tMadison County\tH1\n35805\t1089\tHuntsville\tAL\tMadison County\tH1\n35802\t1089\tHuntsville\tAL\tMadison County\tH1\n35824\t1089\tHuntsville\tAL\tMadison County\tH1\n35750\t1089\tHazel green\tAL\tMadison County\tH1\n35756\t1089\tMadison\tAL\tMadison County\tH1\n35757\t1089\tMadison\tAL\tMadison County\tH1\n35761\t1089\tNew market\tAL\tMadison County\tH1\n35748\t1089\tGurley\tAL\tMadison County\tH1\n35762\t1089\tNormal\tAL\tMadison County\tH1\n35814\t1089\tHuntsville\tAL\tMadison County\tH1\n35899\t1089\tHuntsville\tAL\tMadison County\tH1\n35767\t1089\tRyland\tAL\tMadison County\tH1\n35893\t1089\tHuntsville\tAL\tMadison County\tH1\n35815\t1089\tHuntsville\tAL\tMadison County\tH1\n35804\t1089\tHuntsville\tAL\tMadison County\tH1\n35807\t1089\tHuntsville\tAL\tMadison County\tH1\n35759\t1089\tMeridianville\tAL\tMadison County\tH1\n35896\t1089\tHuntsville\tAL\tMadison County\tH1\n35898\t1089\tHuntsville\tAL\tMadison County\tH1\n35809\t1089\tHuntsville\tAL\tMadison County\tH1\n35806\t1089\tHuntsville\tAL\tMadison County\tH1\n35758\t1089\tMadison\tAL\tMadison County\tH1\n35813\t1089\tHuntsville\tAL\tMadison County\tH1\n36722\t1091\tArlington\tAL\tMarengo County\tH1\n36748\t1091\tLinden\tAL\tMarengo County\tH1\n36745\t1091\tJefferson\tAL\tMarengo County\tH1\n36786\t1091\tUniontown\tAL\tMarengo County\tH1\n36736\t1091\tDixons mills\tAL\tMarengo County\tH1\n36751\t1091\tLower peach tree\tAL\tMarengo County\tH1\n36773\t1091\tSafford\tAL\tMarengo County\tH1\n36783\t1091\tThomaston\tAL\tMarengo County\tH1\n36728\t1091\tCatherine\tAL\tMarengo County\tH1\n36769\t1091\tPine hill\tAL\tMarengo County\tH1\n36784\t1091\tThomasville\tAL\tMarengo County\tH1\n36763\t1091\tMyrtlewood\tAL\tMarengo County\tH1\n36732\t1091\tDemopolis\tAL\tMarengo County\tH1\n36782\t1091\tSweet water\tAL\tMarengo County\tH1\n36764\t1091\tNanafalia\tAL\tMarengo County\tH1\n36742\t1091\tGallion\tAL\tMarengo County\tH1\n36738\t1091\tFaunsdale\tAL\tMarengo County\tH1\n36754\t1091\tMagnolia\tAL\tMarengo County\tH1\n36904\t1091\tButler\tAL\tMarengo County\tH1\n35554\t1093\tEldridge\tAL\tMarion County\tH1\n35594\t1093\tWinfield\tAL\tMarion County\tH1\n35593\t1093\tVina\tAL\tMarion County\tH1\n35581\t1093\tPhil campbell\tAL\tMarion County\tH1\n35565\t1093\tHaleyville\tAL\tMarion County\tH1\n35563\t1093\tGuin\tAL\tMarion County\tH1\n35564\t1093\tHackleburg\tAL\tMarion County\tH1\n35570\t1093\tHamilton\tAL\tMarion County\tH1\n35548\t1093\tBrilliant\tAL\tMarion County\tH1\n35552\t1093\tDetroit\tAL\tMarion County\tH1\n35571\t1093\tHodges\tAL\tMarion County\tH1\n35543\t1093\tBear creek\tAL\tMarion County\tH1\n35175\t1095\tUnion grove\tAL\tMarshall County\tH1\n35760\t1095\tNew hope\tAL\tMarshall County\tH1\n35980\t1095\tHorton\tAL\tMarshall County\tH1\n35776\t1095\tWoodville\tAL\tMarshall County\tH1\n35950\t1095\tAlbertville\tAL\tMarshall County\tH1\n35769\t1095\tScottsboro\tAL\tMarshall County\tH1\n35975\t1095\tGroveoak\tAL\tMarshall County\tH1\n35087\t1095\tJoppa\tAL\tMarshall County\tH1\n35957\t1095\tBoaz\tAL\tMarshall County\tH1\n35031\t1095\tBlountsville\tAL\tMarshall County\tH1\n35951\t1095\tAlbertville\tAL\tMarshall County\tH1\n35956\t1095\tBoaz\tAL\tMarshall County\tH1\n35976\t1095\tGuntersville\tAL\tMarshall County\tH1\n35747\t1095\tGrant\tAL\tMarshall County\tH1\n35016\t1095\tArab\tAL\tMarshall County\tH1\n35754\t1095\tLaceys spring\tAL\tMarshall County\tH1\n35952\t1095\tAltoona\tAL\tMarshall County\tH1\n35962\t1095\tCrossville\tAL\tMarshall County\tH1\n35755\t1095\tLangston\tAL\tMarshall County\tH1\n35964\t1095\tDouglas\tAL\tMarshall County\tH1\n36571\t1097\tSaraland\tAL\tMobile County\tH1\n36695\t1097\tMobile\tAL\tMobile County\tH1\n36587\t1097\tWilmer\tAL\tMobile County\tH1\n36613\t1097\tEight mile\tAL\tMobile County\tH1\n36663\t1097\tMobile\tAL\tMobile County\tH1\n36652\t1097\tMobile\tAL\tMobile County\tH1\n36528\t1097\tDauphin island\tAL\tMobile County\tH1\n36525\t1097\tCreola\tAL\tMobile County\tH1\n36582\t1097\tTheodore\tAL\tMobile County\tH1\n36572\t1097\tSatsuma\tAL\tMobile County\tH1\n36612\t1097\tMobile\tAL\tMobile County\tH1\n36689\t1097\tMobile\tAL\tMobile County\tH1\n36618\t1097\tMobile\tAL\tMobile County\tH1\n36603\t1097\tMobile\tAL\tMobile County\tH1\n36608\t1097\tMobile\tAL\tMobile County\tH1\n36560\t1097\tMount vernon\tAL\tMobile County\tH1\n36604\t1097\tMobile\tAL\tMobile County\tH1\n36617\t1097\tMobile\tAL\tMobile County\tH1\n36640\t1097\tMobile\tAL\tMobile County\tH1\n36505\t1097\tAxis\tAL\tMobile County\tH1\n36509\t1097\tBayou la batre\tAL\tMobile County\tH1\n36521\t1097\tChunchula\tAL\tMobile County\tH1\n36575\t1097\tSemmes\tAL\tMobile County\tH1\n36607\t1097\tMobile\tAL\tMobile County\tH1\n36606\t1097\tMobile\tAL\tMobile County\tH1\n36609\t1097\tMobile\tAL\tMobile County\tH1\n36544\t1097\tIrvington\tAL\tMobile County\tH1\n36619\t1097\tMobile\tAL\tMobile County\tH1\n36685\t1097\tMobile\tAL\tMobile County\tH1\n36691\t1097\tMobile\tAL\tMobile County\tH1\n36601\t1097\tMobile\tAL\tMobile County\tH1\n36671\t1097\tMobile\tAL\tMobile County\tH1\n36512\t1097\tBucks\tAL\tMobile County\tH1\n36523\t1097\tCoden\tAL\tMobile County\tH1\n36605\t1097\tMobile\tAL\tMobile County\tH1\n36693\t1097\tMobile\tAL\tMobile County\tH1\n36602\t1097\tMobile\tAL\tMobile County\tH1\n36644\t1097\tMobile\tAL\tMobile County\tH1\n36610\t1097\tMobile\tAL\tMobile County\tH1\n36660\t1097\tMobile\tAL\tMobile County\tH1\n36688\t1097\tMobile\tAL\tMobile County\tH1\n36615\t1097\tMobile\tAL\tMobile County\tH1\n36616\t1097\tMobile\tAL\tMobile County\tH1\n36633\t1097\tMobile\tAL\tMobile County\tH1\n36541\t1097\tGrand bay\tAL\tMobile County\tH1\n36611\t1097\tMobile\tAL\tMobile County\tH1\n36670\t1097\tMobile\tAL\tMobile County\tH1\n36568\t1097\tSaint elmo\tAL\tMobile County\tH1\n36675\t1097\tMobile\tAL\tMobile County\tH1\n36522\t1097\tCitronelle\tAL\tMobile County\tH1\n36590\t1097\tTheodore\tAL\tMobile County\tH1\n36444\t1099\tFranklin\tAL\tMonroe County\tH1\n36502\t1099\tAtmore\tAL\tMonroe County\tH1\n36481\t1099\tVredenburgh\tAL\tMonroe County\tH1\n36439\t1099\tExcel\tAL\tMonroe County\tH1\n36751\t1099\tLower peach tree\tAL\tMonroe County\tH1\n36425\t1099\tBeatrice\tAL\tMonroe County\tH1\n36033\t1099\tGeorgiana\tAL\tMonroe County\tH1\n36726\t1099\tCamden\tAL\tMonroe County\tH1\n36471\t1099\tPeterman\tAL\tMonroe County\tH1\n36458\t1099\tMexia\tAL\tMonroe County\tH1\n36460\t1099\tMonroeville\tAL\tMonroe County\tH1\n36401\t1099\tEvergreen\tAL\tMonroe County\tH1\n36475\t1099\tRepton\tAL\tMonroe County\tH1\n36482\t1099\tWhatley\tAL\tMonroe County\tH1\n36470\t1099\tPerdue hill\tAL\tMonroe County\tH1\n36445\t1099\tFrisco city\tAL\tMonroe County\tH1\n36480\t1099\tUriah\tAL\tMonroe County\tH1\n36768\t1099\tPine apple\tAL\tMonroe County\tH1\n36043\t1101\tHope hull\tAL\tMontgomery County\tH1\n36108\t1101\tMontgomery\tAL\tMontgomery County\tH1\n36029\t1101\tFitzpatrick\tAL\tMontgomery County\tH1\n36112\t1101\tMontgomery\tAL\tMontgomery County\tH1\n36052\t1101\tMathews\tAL\tMontgomery County\tH1\n36102\t1101\tMontgomery\tAL\tMontgomery County\tH1\n36069\t1101\tRamer\tAL\tMontgomery County\tH1\n36104\t1101\tMontgomery\tAL\tMontgomery County\tH1\n36013\t1101\tCecil\tAL\tMontgomery County\tH1\n36111\t1101\tMontgomery\tAL\tMontgomery County\tH1\n36124\t1101\tMontgomery\tAL\tMontgomery County\tH1\n36103\t1101\tMontgomery\tAL\tMontgomery County\tH1\n36047\t1101\tLetohatchee\tAL\tMontgomery County\tH1\n36115\t1101\tMontgomery\tAL\tMontgomery County\tH1\n36113\t1101\tMontgomery\tAL\tMontgomery County\tH1\n36110\t1101\tMontgomery\tAL\tMontgomery County\tH1\n36125\t1101\tMontgomery\tAL\tMontgomery County\tH1\n36101\t1101\tMontgomery\tAL\tMontgomery County\tH1\n36130\t1101\tMontgomery\tAL\tMontgomery County\tH1\n36114\t1101\tMontgomery\tAL\tMontgomery County\tH1\n36118\t1101\tMontgomery\t
